vi "niRFUtil WFM Remove Frequency Offset - Coarse.vi"(0 "Waveform In":T1 {"y" format="%.2f"; "dx" format="%^.2e"; "x0" format="%^.2e"}, 5 "Reference Waveform In":T1 {"y" format="%.2f"; "dx" format="%^.2e"; "x0" format="%^.2e"}) -> (4 "Waveform Out":T1 {"y" format="%.2f"; "dx" format="%^.2e"; "x0" format="%^.2e"}, 6 "Reference Waveform Out":T1 {"y" format="%.2f"; "dx" format="%^.2e"; "x0" format="%^.2e"}, 13 "Offset, Hz":sgl format="%^.2e")   [LabVIEW 2015, in "niRFUtil.lvlib"]
doc: "(c) Copyright 2006, National Instruments, Inc. This VI may not be duplicated, sold, or distributed without written consent from National Instruments."
uses:
  niRFUtil.lvlib
  Includes/niRFUtil INC Complex Waveform.ctl
  Includes/niRFUtil INC Complex Array.ctl
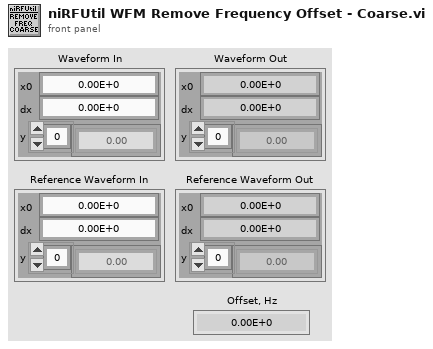
[diagram p1: front panel]
types:
  T1 = typedef "niRFUtil.lvlib/niRFUtil INC Complex Waveform.ctl" = cluster{"x0":dbl, "dx":dbl, "y":T2}
  T2 = typedef "niRFUtil.lvlib/niRFUtil INC Complex Array.ctl" = csg[]
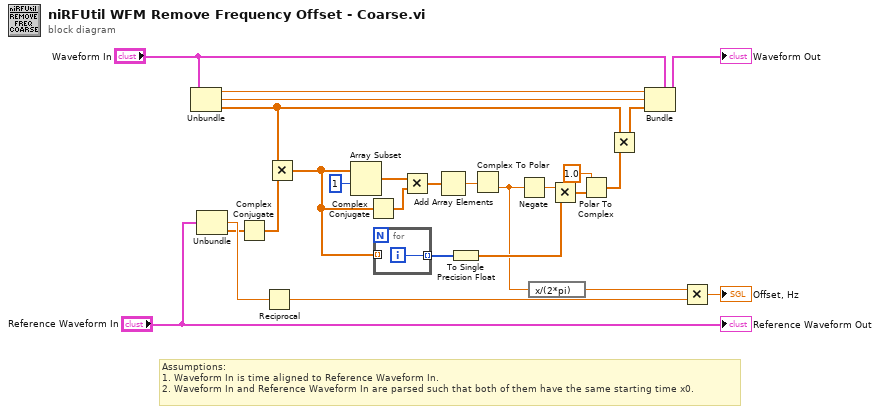
[diagram p0: block diagram]
diagram:
  # "Assumptions:\n1. Waveform In is time aligned to Reference Waveform In.\n2. Waveform In and Reference Waveform In are parsed such that both of them have the same starting time x0."
  n1 = Unbundle("Waveform In") -> ("x0"=w8:dbl, "dx"=w9:dbl, "y"=w12:T2)
  n2 = Unbundle("Reference Waveform In") -> ("dx"=w23:dbl, "y"=w19:T2)  [unwired: 1 out]
  n3 = Complex Conjugate(1:w19) -> (0:w26:T2)
  n4 = Reciprocal(x=w23) -> (1/x=w22:dbl)
  n5 = Multiply(x=w12, y=w26) -> (x*y=w1:T2)
  n6 = Array Subset(array=w1, index=1) -> (w16:T2)  [unwired: 1 in]
  n7 = Complex Conjugate(1:w1) -> (0:w18:T2)
  n8 = for {
    tunnel: [w27] -> w6 mode=indexing
    tunnel: w1 -> [_] mode=indexing
    i -> [w27]
  }
  n9 = Multiply(x=w16, y=w18) -> (x*y=w4:T2)
  n10 = Add Array Elements(numeric array=w4) -> (sum=w3:csg)
  n11 = To Single Precision Float(number=w6) -> (single precision float=w5:sgl[])
  n12 = Complex To Polar(r * e^(i*theta)=w3) -> (theta=w2:sgl)  [unwired: 1 out]
  n13 = Negate(x=w2) -> (-x=w15:sgl)
  n14 = expression code="x/(2*pi)"(w2) -> (w24:sgl)
  n15 = Multiply(x=w15, y=w5) -> (x*y=w14:sgl[])
  n16 = Polar To Complex(1:w14, 2:sgl 1.0) -> (0:w11:csg[])
  n17 = Multiply(x=w12, y=w11) -> (x*y=w10:T2)
  n18 = Bundle(cluster="Waveform In", "x0"=w8, "dx"=w9, "y"=w10) -> (→"Waveform Out":T1)
  n19 = Multiply(x=w24, y=w22) -> (x*y=→"Offset, Hz":dbl)
  "Reference Waveform Out" <- "Reference Waveform In"
